vi "Add Sequence Number and CRC.vi"(8 "Error In":errorcluster, 11 "Message In":string) -> (0 "Error Out":errorcluster, 3 "MAVLink Message Out":string)   [LabVIEW 2014]
uses:
  CRC/MAVLink CRC v2 Generate.vi
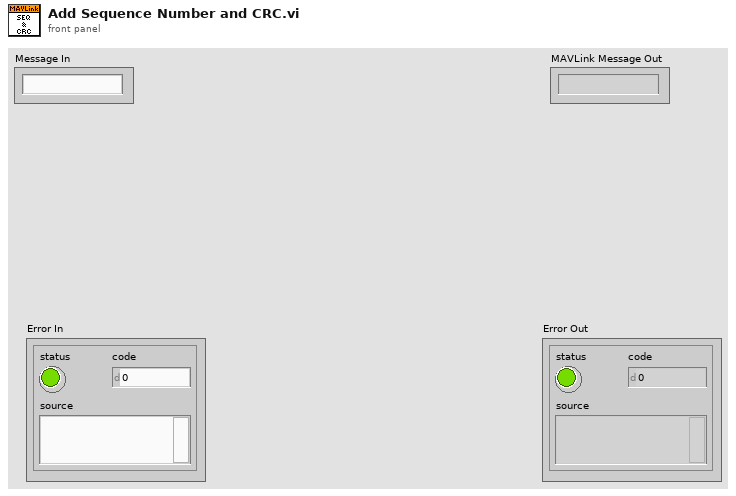
[diagram p1: front panel]
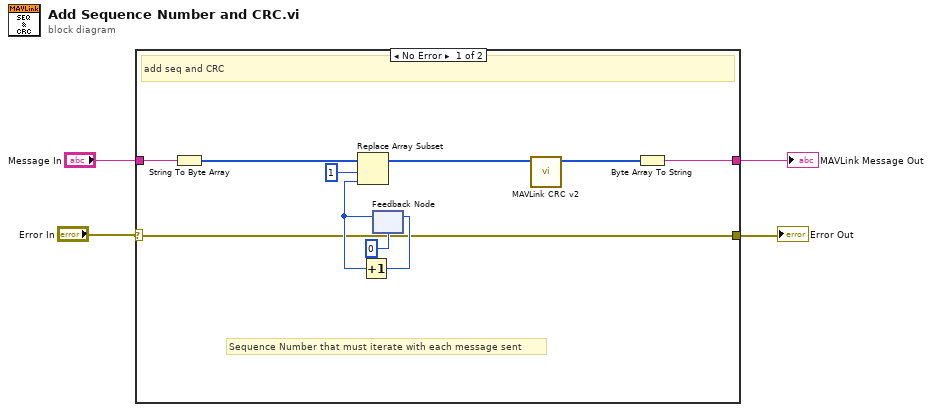
[diagram p0: block diagram]
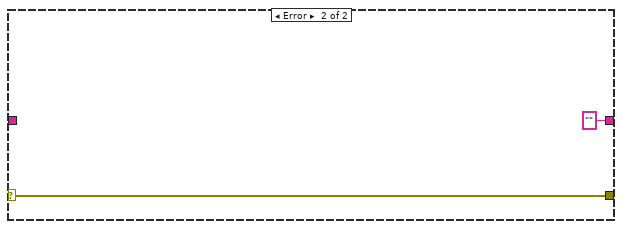
[diagram p2: hidden frame]
diagram:
  n1 = case shown="No Error" "Error In" {
    selector: "Error In" -> [w5 w16]
    tunnel: "Message In" -> [w8 _]
    tunnel: [w6 "" ("string")] -> w3
    tunnel: [w5 w16] -> w1
    frame No Error {
      # "Sequence Number that must iterate with each message sent"
      # "add seq and CRC"
      n2 = String To Byte Array(string=w8) -> (unsigned byte array=w7:u8[])
      n3 = feedback #1(u8 0) -> (w13:u8)
      n4 = Replace Array Subset(array=w7, new element=w13, index=1) -> (w10:u8[])
      n5 = Increment(x=w13) -> (x+1=w14:u8)
      n6 = feedback-in #1(w14) -> ()
      n7 = call-poly "MAVLink CRC v2.vi"("Message"=w10) -> ("Message w/ CRC"=w9:u8[])  [unwired: 10 in]
      n8 = Byte Array To String(unsigned byte array=w9) -> (string=w6:string)
    }
    frame Error {
    }
  }
  "MAVLink Message Out" <- w3
  "Error Out" <- w1
